vi "Variable@VariableSave__Parameter.vi"(1 "ParamterIn":string) -> (0 "ParamterOut":string)   [LabVIEW 2019]
uses:
  MainFrame/Global.vi
panel:
  in  "VariableList":string(combo)
  in  "FileName":string(combo)
  in  "Confirm":bool
  # "Variable@VariableSave $VariableFile(,Variable1,Variable2......)"
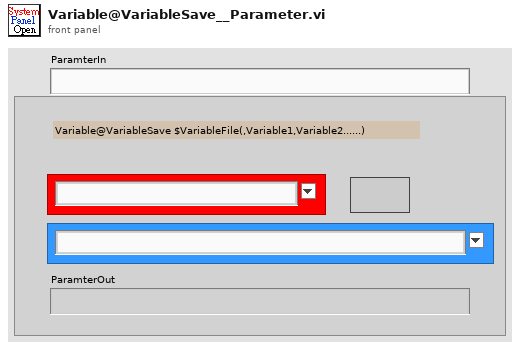
[diagram p1: front panel]
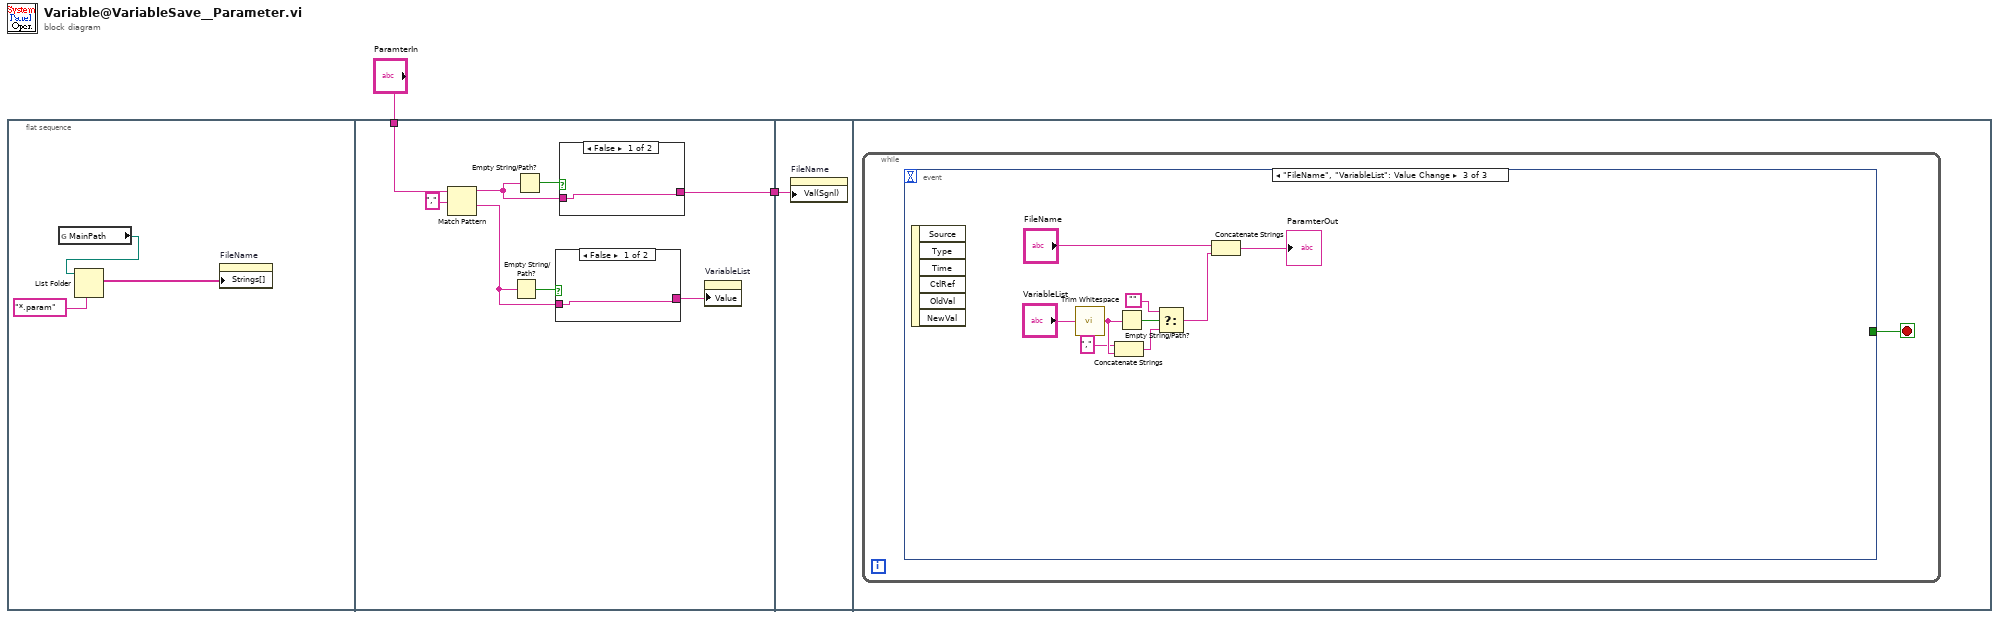
[diagram p0: block diagram]
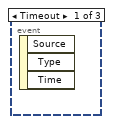
[diagram p4: hidden frame]
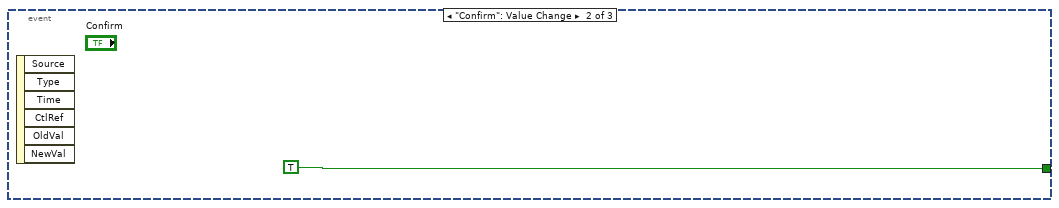
[diagram p5: hidden frame]
diagram:
  n1 = flat-sequence {
    tunnel: "ParamterIn" -> [w11]
    tunnel: [w12] -> w1
    tunnel: w1 -> [w18]
    frame #0 {
      n2 = global read "Global.vi" "MainPath"() -> (w5:path)
      n3 = List Folder(path=w5, pattern="*.param") -> (filenames=w3:string[])  [unwired: 2 in, 3 out]
      n4 = property on="FileName" class="CmbBox"("Strings[]"=w3) -> ()  [unwired: 2 in, 2 out]
    }
    frame #1 {
      n5 = Match Pattern(string=w11, regular expression=",") -> (before substring=w9:string, after substring=w7:string)  [unwired: 1 in, 2 out]
      n6 = Empty String/Path?(string/path=w7) -> (empty?=w8:bool)
      n7 = Empty String/Path?(string/path=w9) -> (empty?=w13:bool)
      n8 = case shown="False" w8 {
        tunnel: w7 -> [w14 w15]
        tunnel: [w14 w15] -> w6
        frame False {
        }
        frame True {
        }
      }
      n9 = case shown="False" w13 {
        tunnel: w9 -> [w16 w17]
        tunnel: [w16 w17] -> w12
        frame False {
        }
        frame True {
        }
      }
      n10 = property on="VariableList" class="CmbBox"("Value"=w6) -> ()  [unwired: 2 in, 2 out]
    }
    frame #2 {
      n11 = property on="FileName" class="CmbBox"("Val(Sgnl)"=w18) -> ()  [unwired: 2 in, 2 out]
    }
    frame #3 {
      n12 = while {
        stop <- w19 stop-if-true
        n13 = event shown="[2] \"FileName\", \"VariableList\": Value Change" {
          selector: _ -> [_ _ _]
          dyn-events: _ -> [_ _ _]
          timeout: _ -> [_ _ _]
          tunnel: [_ TRUE _] -> w19
          event Timeout {
            n14 = event-data() -> ()  [unwired: 1 in, 3 out]
          }
          event "Confirm": Value Change {
            n15 = event-data() -> ()  [unwired: 1 in, 6 out]
          }
          event "FileName", "VariableList": Value Change {
            n16 = event-data() -> ()  [unwired: 1 in, 6 out]
            n17 = call <vilib>:"Trim Whitespace.vi"("string"="VariableList") -> ("trimmed string"=w26:string)  [unwired: 1 in]
            n18 = Concatenate Strings("," ("string"), w26) -> (w24:string)
            n19 = Empty String/Path?(string/path=w26) -> (empty?=w28:bool)
            n20 = Select(t="", s=w28, f=w24) -> (s? t:f=w22:string)
            n21 = Concatenate Strings("FileName", w22) -> (→"ParamterOut":string)
          }
        }
      }
    }
  }
